vi "Resolve Replicates.vi"(6 "Teams in":refnum<class "Team.lvclass">[](array[class]), 7 "Round":u32, 9 "New Map in":refnum<class "Map.lvclass">, 11 "Map in":refnum<class "Map.lvclass">) -> (1 "New Map out":refnum<class "Map.lvclass">, 4 "Teams out":refnum<class "Team.lvclass">[](array[class]))   [LabVIEW 2020]
uses:
  Map.lvclass
  Team/Team.lvclass
  Map.lvclass/Map.ctl
  Position.ctl
  Action.ctl
  Team/Team.lvclass/Team.ctl
  Square/Square.lvclass/Square.ctl
  Square/Square.lvclass
  Direction Position Offsets.vi
  Normalize Position.vi
  Team/Team Index.vi
  Team/Add Turn Stats.vi
  SquareBattle.lvlib
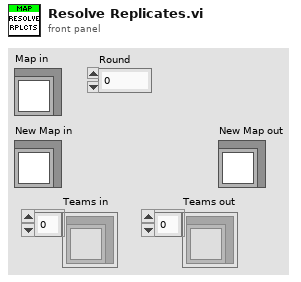
[diagram p1: front panel]
types:
  T1 = typedef "SquareBattle.lvlib/Position.ctl" = cluster{"Row":i32, "Col":i32}
  T2 = typedef "SquareBattle.lvlib/Action.ctl" = enum16{"Wait", "Move", "Attack", "Replicate"}
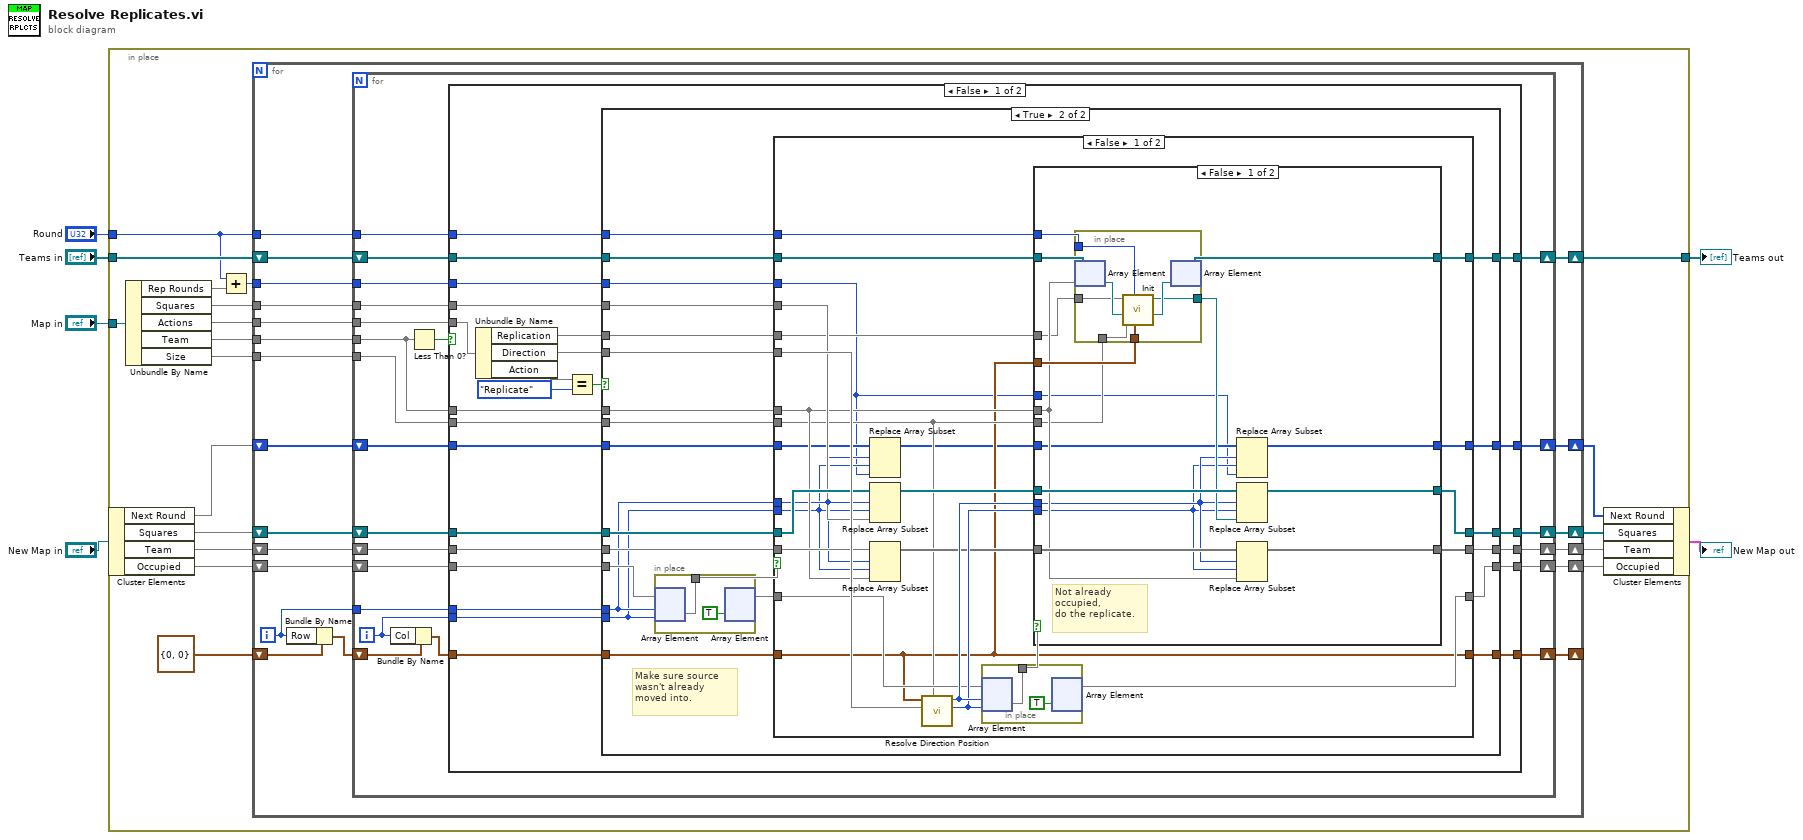
[diagram p0: block diagram]
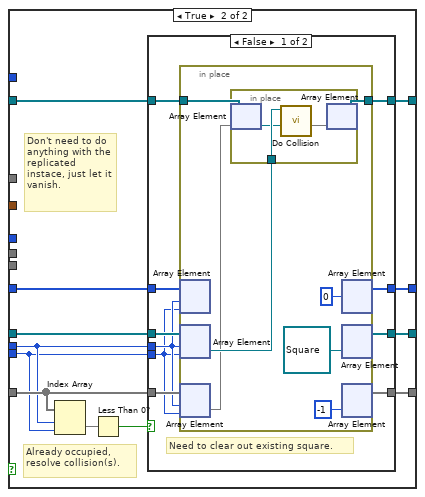
[diagram p3: hidden frame]
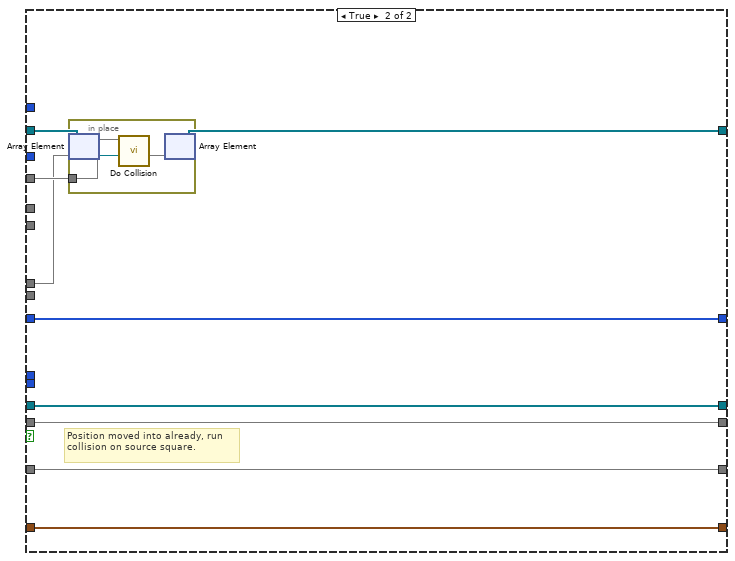
[diagram p5: hidden frame]
diagram:
  n1 = in-place {
    in-place-border: "Map in" -> [w25]
    in-place-border: "Teams in" -> [w13]
    in-place-border: [w12] -> w4
    in-place-border: "Round" -> [w8]
    n2 = in-place-cluster #1("New Map in") -> ("Next Round"=w11, "Squares"=w21, "Team"=w20, "Occupied"=w19)
    n3 = Unbundle By Name(w25) -> ("Rep Rounds"=w9, "Squares"=w24, "Actions"=w23, "Team"=w22, "Size"=w14)
    n4 = Add(x=w8, y=w9) -> (x+y=w7:u32)
    n5 = for {
      tunnel: w24 -> [w45]
      tunnel: w23 -> [w44]
      tunnel: w22 -> [w43]
      shift-right: [w37] -> w18
      shift-left: w21 -> [w42]
      shift-right: [w39] -> w17
      shift-left: w19 -> [w40]
      shift-right: [w38] -> w16
      shift-left: w20 -> [w41]
      tunnel: w14 -> [w36]
      shift-right: [w33] -> _
      shift-left: T1 {"Row"=0, "Col"=0} ("Position") -> [w35]
      shift-right: [w31] -> w12
      shift-left: w13 -> [w32]
      tunnel: w8 -> [w29]
      shift-right: [w27] -> w10
      shift-left: w11 -> [w28]
      tunnel: w7 -> [w26]
      i -> [w30]
      n6 = Bundle By Name(cluster=w35, "Row"=w30) -> (w34:T1)
      n7 = for {
        tunnel: w45 -> [w64]
        tunnel: w44 -> [w65]
        tunnel: w43 -> [w66]
        shift-right: [w63] -> w37
        shift-left: w42 -> [w62]
        shift-right: [w59] -> w39
        shift-left: w40 -> [w58]
        shift-right: [w61] -> w38
        shift-left: w41 -> [w60]
        tunnel: w36 -> [w55]
        shift-right: [w54] -> w33
        shift-left: w34 -> [w57]
        shift-right: [w52] -> w31
        shift-left: w32 -> [w53]
        tunnel: w30 -> [w51]
        tunnel: w29 -> [w49]
        shift-right: [w47] -> w27
        shift-left: w28 -> [w48]
        tunnel: w26 -> [w46]
        i -> [w50]
        n8 = Bundle By Name(cluster=w57, "Col"=w50) -> (w56:T1)
        n9 = Less Than 0?(x=w66) -> (x < 0?=w67:bool)
        n10 = case shown="False" w67 {
          tunnel: w66 -> [w80 _]
          tunnel: w65 -> [w92 _]
          tunnel: w64 -> [w89 _]
          tunnel: [w86 w229] -> w63
          tunnel: w62 -> [w85 w229]
          tunnel: [w84 w228] -> w61
          tunnel: w60 -> [w83 w228]
          tunnel: [w82 w227] -> w59
          tunnel: w58 -> [w81 w227]
          tunnel: w56 -> [w79 w226]
          tunnel: w55 -> [w78 _]
          tunnel: [w77 w226] -> w54
          tunnel: w53 -> [w76 w225]
          tunnel: [w75 w225] -> w52
          tunnel: w51 -> [w73 _]
          tunnel: w50 -> [w72 _]
          tunnel: w49 -> [w71 _]
          tunnel: w48 -> [w70 w224]
          tunnel: [w69 w224] -> w47
          tunnel: w46 -> [w68 _]
          frame False {
            n11 = Unbundle By Name(w92) -> ("Replication"=w74, "Direction"=w88, "Action"=w91)
            n12 = Equal?(x=w91, y=Action."Replicate") -> (x = y?=w87:bool)
            n13 = case shown="True" w87 {
              tunnel: w89 -> [_ w107]
              tunnel: w88 -> [_ w121]
              tunnel: [w98 w114] -> w86
              tunnel: w85 -> [w98 w117]
              tunnel: [w97 w115] -> w84
              tunnel: w83 -> [w97 w118]
              tunnel: [w96 w119] -> w82
              tunnel: w81 -> [w96 w110]
              tunnel: w80 -> [_ w116]
              tunnel: w79 -> [w95 w111]
              tunnel: w78 -> [_ w120]
              tunnel: [w95 w102] -> w77
              tunnel: w76 -> [w94 w113]
              tunnel: [w94 w112] -> w75
              tunnel: w74 -> [_ w106]
              tunnel: w73 -> [_ w105]
              tunnel: w72 -> [_ w104]
              tunnel: w71 -> [_ w103]
              tunnel: w70 -> [w93 w101]
              tunnel: [w93 w100] -> w69
              tunnel: w68 -> [_ w99]
              frame False {
                # "Not a replicate, do nothing."
              }
              frame True {
                # "Make sure source wasn't already moved into."
                n14 = in-place {
                  in-place-border: [w223] -> w108
                  n15 = in-place-array #2(w110, w105, w104) -> (w223)
                  n16 = in-place-array #2(TRUE ("element")) -> (w109)  [unwired: 2 out]
                }
                n17 = case shown="False" w108 {
                  tunnel: w121 -> [w147 _]
                  tunnel: w120 -> [w132 _]
                  tunnel: [w146 w218] -> w119
                  tunnel: w118 -> [w136 w217]
                  tunnel: w117 -> [w139 w216]
                  tunnel: w116 -> [w135 w210]
                  tunnel: [w144 w217] -> w115
                  tunnel: [w143 w216] -> w114
                  tunnel: w113 -> [w133 w215]
                  tunnel: [w130 w213] -> w112
                  tunnel: w111 -> [w129 w212]
                  tunnel: w109 -> [w140 w218]
                  tunnel: w107 -> [w138 w214]
                  tunnel: w106 -> [w131 _]
                  tunnel: w105 -> [w126 _]
                  tunnel: w104 -> [w125 _]
                  tunnel: w103 -> [w128 _]
                  tunnel: [w129 w212] -> w102
                  tunnel: w101 -> [w127 w211]
                  tunnel: [w122 w211] -> w100
                  tunnel: w99 -> [w124 _]
                  frame False {
                    n18 = Replace Array Subset(array=w127, new element=w124, index (row)=w126, index (col)=w125) -> (w123:u32[])
                    n19 = Replace Array Subset(array=w139, new element=w138, index (row)=w126, index (col)=w125) -> (w137:refnum<class "Square.lvclass">[])
                    n20 = Replace Array Subset(array=w136, new element=w135, index (row)=w126, index (col)=w125) -> (w134:void[])
                    n21 = call "Resolve Direction Position.vi"("Board Size"=w132, "Direction"=w147, "From"=w129) -> ("Col"=w141:i32, "Row"=w142:i32)  [unwired: 6 in, 1 out]
                    n22 = in-place {
                      in-place-border: [w209] -> w145
                      n23 = in-place-array #3(w140, w142, w141) -> (w209)
                      n24 = in-place-array #3(TRUE ("element")) -> (w146)  [unwired: 2 out]
                    }
                    n25 = case shown="False" w145 {
                      tunnel: w134 -> [w164 w178]
                      tunnel: w137 -> [w162 w181]
                      tunnel: w135 -> [w158 _]
                      tunnel: [w163 w179] -> w144
                      tunnel: [w161 w180] -> w143
                      tunnel: w142 -> [w151 w177]
                      tunnel: w141 -> [w150 w176]
                      tunnel: [w159 w175] -> w130
                      tunnel: w129 -> [w160 _]
                      tunnel: w133 -> [w157 w174]
                      tunnel: w132 -> [w156 _]
                      tunnel: w131 -> [w155 _]
                      tunnel: w128 -> [w154 _]
                      tunnel: w124 -> [w149 _]
                      tunnel: w123 -> [w152 w173]
                      tunnel: [w148 w172] -> w122
                      frame False {
                        # "Not already occupied,\ndo the replicate."
                        n26 = in-place {
                          in-place-border: w160 -> [w167]
                          in-place-border: w156 -> [w169]
                          in-place-border: w155 -> [w168]
                          in-place-border: w154 -> [w166]
                          in-place-border: [w165] -> w153
                          n27 = in-place-array #4(w157, w158) -> (w171:refnum<class "Team.lvclass">)
                          n28 = call "Init.vi"("Position"=w167, "Round"=w166, "Team in"=w171, "Board Size"=w169, "Square in"=w168) -> ("Team out"=w170:refnum<class "Team.lvclass">, "Square out"=w165:refnum<class "Square.lvclass">)  [unwired: 5 in]
                          n29 = in-place-array #4(w170) -> (w159:refnum<class "Team.lvclass">[])  [unwired: 1 out]
                        }
                        n30 = Replace Array Subset(array=w152, new element=w149, index (row)=w151, index (col)=w150) -> (w148:u32[])
                        n31 = Replace Array Subset(array=w162, new element=w153, index (row)=w151, index (col)=w150) -> (w161:refnum<class "Square.lvclass">[])
                        n32 = Replace Array Subset(array=w164, new element=w158, index (row)=w151, index (col)=w150) -> (w163:void[])
                      }
                      frame True {
                        # "Don't need to do anything with the replicated instace, just let it vanish."
                        # "Already occupied, resolve collision(s)."
                        n33 = Index Array(array=w178, index (row)=w177, index (col)=w176) -> (element=w183)
                        n34 = Less Than 0?(x=w183) -> (x < 0?=w182:bool)
                        n35 = case shown="False" w182 {
                          tunnel: w181 -> [w193 w207]
                          tunnel: [w191 w207] -> w180
                          tunnel: [w188 w206] -> w179
                          tunnel: w178 -> [w190 w206]
                          tunnel: w177 -> [w186 _]
                          tunnel: w176 -> [w185 _]
                          tunnel: w174 -> [w192 w205]
                          tunnel: [w189 w205] -> w175
                          tunnel: w173 -> [w187 w204]
                          tunnel: [w184 w204] -> w172
                          frame False {
                            # "Need to clear out existing square."
                            n36 = in-place {
                              in-place-border: w192 -> [w195]
                              in-place-border: [w197] -> w189
                              n37 = in-place-array #5(w187, w186, w185) -> ()  [unwired: 1 out]
                              n38 = in-place-array #6(w193, w186, w185) -> (w198:refnum<class "Square.lvclass">)
                              n39 = in-place-array #7(w190, w186, w185) -> (w196)
                              n40 = in-place {
                                in-place-border: w198 -> [w203]
                                n41 = in-place-array #8(w195, w196) -> (w201:refnum<class "Team.lvclass">)
                                n42 = call "Do Collision.vi"(9:w201, "Square"=w203) -> (1:w202)  [unwired: 8 in, 1 out]
                                n43 = in-place-array #8(w202) -> (w197:refnum<class "Team.lvclass">[])  [unwired: 1 out]
                              }
                              n44 = in-place-array #5(u32 0 ("element")) -> (w184:u32[])  [unwired: 2 out]
                              n45 = in-place-array #6(refnum<class "Square.lvclass"> refnum ("element")) -> (w191:refnum<class "Square.lvclass">[])  [unwired: 2 out]
                              n46 = in-place-array #7(-1 ("element")) -> (w188:void[])  [unwired: 2 out]
                            }
                          }
                          frame True {
                            # "Already emptied, don't need to handle collision for target."
                          }
                        }
                      }
                    }
                  }
                  frame True {
                    # "Position moved into already, run collision on source square."
                    n47 = in-place {
                      in-place-border: w214 -> [w219]
                      n48 = in-place-array #9(w215, w210) -> (w221:refnum<class "Team.lvclass">)
                      n49 = call "Do Collision.vi"(9:w221, "Square"=w219) -> (1:w220)  [unwired: 8 in, 1 out]
                      n50 = in-place-array #9(w220) -> (w213:refnum<class "Team.lvclass">[])  [unwired: 1 out]
                    }
                  }
                }
              }
            }
          }
          frame True {
            # "Empty, do nothing."
          }
        }
      }
    }
    n51 = in-place-cluster #1("Next Round"=w10, "Squares"=w18, "Team"=w16, "Occupied"=w17) -> (→"New Map out":cluster{})
  }
  "Teams out" <- w4
